vi "NIFPGA-MCS.get bin data.vi"(0 "i ref in":refnum<vi>, 3 "ms timeout (10000)":i32=10000, 5 "error in (no error)":errorcluster) -> (14 "i ref out":refnum<vi>, 16 "Output Waveform":waveform(dbl), 19 "error out":errorcluster)   [LabVIEW 2014, in "NIFPGA-MCS.lvlib"]
doc: "Reads the previously acquired data from the device."
uses:
  NIFPGA-MCS.lvlib
  CSCore/CSApplicationBaseClasses/MCSBase/MCSBase.directionType.ctl
  CSCore/CSApplicationBaseClasses/MCSBase/MCSBase.serviceType.ctl
  CSlibraries/UtilityLib/UtilityLib.valueStatus.ctl
  CSCore/CSApplicationBaseClasses/DeviceBase/DeviceBase.deviceState.ctl
  CSCore/CSSystem/CoreDefs/CoreDefs.error_type.ctl
  CSCore/CSSystem/CoreDefs/CoreDefs.error_severity.ctl
  CSCore/CSApplicationBaseClasses/MCSBase/MCSBase.lvlib
  CSlibraries/UtilityLib/UtilityLib.lvlib
  CSCore/CSApplicationBaseClasses/DeviceBase/DeviceBase.lvlib
  CSCore/CSSystem/CoreLib/CoreLib.lvlib
  CSinstr.lib/NI-FPGA-MCS/host/instrumentDriver/NI-FPGA-MCS_Driver.lvlib
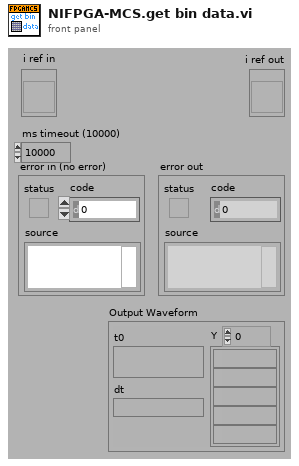
[diagram p1: front panel]
types:
  T1 = typedef "MCSBase.lvlib/MCSBase.serviceType.ctl" = enum16{"counts", "totalCounts", "binWidth", "nOfBins", "nOfRecords", "status", "discrLevel", "discrSlope", "triggerLevel", "triggerSlope"}
  T2 = typedef "UtilityLib.lvlib/UtilityLib.valueStatus.ctl" = enum16{"no info available", "stand by/off", "on", "warning", "alarm/malfunction", "not implemented", "user action required", "important information", "system default", "control default", "indicator default", "button default"}
  T3 = typedef "CoreDefs.error_severity.ctl" = enum16{"undefined", "information", "warning", "error", "fatal"}
  T4 = typedef "CoreDefs.error_type.ctl" = enum16{"no error", "can't load process", "can't unload process", "process does not exist", "can't install process", "can't remove process", "unknown function", "time out", "can't execute function", "duplicate queue name", "super not found", "caller queue invalid", "can't ping process", "unknown error", "VISA Error", "VISA timeout", "GPIB timeout", "GPIB error", "communication error", "data type mismatch", "can't read data from OPC server", "can't write data to OPC server", "OET error", "function not implemented", "process already exists", "invalid Shared Variable name", "error writing Shared Variable", "error reading Shared Variable", "invalid client name", "corrupt database", "unknown class", "call not authorized", "parameter out of range", "OET timeout: can't get data to modify", "invalid queue name", "requested operation incompatible with current state", "event undefined", "event disabled", "state undefined", "caller is not a friend", "EventBuilder: bad eventID", "EventBuilder: no DAQ devices", "a thread must not stop itself", "UNUSED ELEMENT4", "DiscArchiver: eventData incomplete", "DiscArchiver: eventData does not belong to run", "DiscArchiver: can't open file", "DiscArchiver: can't write to file", "DiscArchiver: available disc space low", "can't acquire semaphore", "error reading data from database", "notifier object is not existing", "can't register process", "can't unregister process", "illegal event type", "object disabled", "object already exists", "can't change state", "Instrument not found", "no connection to remote node", "invalid reference", "N/A", "UNUSED ELEMENT 1", "element not found", "illegal TCP/IP connection detected", "object does not exist", "invalid access ID", "unknown CS system", "invalid privilige", "unsupported data type", "unsupported server type", "IO server already exists", "Shared Variable already exists"}
  T5 = typedef "MCSBase.lvlib/MCSBase.directionType.ctl" = enum16{"unknown", "update actual value", "update nominal value", "update both"}
  T6 = typedef "NIFPGA-MCS.lvlib/NIFPGA-MCS.i attribute.ctl" = cluster{"fpgaViRef":T7}
  T7 = typedef "NI-FPGA-MCS_Driver.lvlib/fpga_vi_ref.ctl" = refnum<k20>
  T8 = typedef "MCSBase.lvlib/MCSBase.i attribute.ctl" = cluster{"actValues":T9, "nomValues":T9}
  T9 = typedef "MCSBase.lvlib/MCSBase.parameters.ctl" = cluster{"counts":i32, "totalCounts":i32, "status":i32, "binWidth [us]":dbl, "nOfBins":i32, "nOfRecords":i32, "discLevel [V]":dbl, "discSlope":bool, "triggerLevel [V]":dbl, "triggerSlope":bool, "serviceIDs":cluster{"countslID":i32, "totalCountsID":i32, "binWidthID":i32, "nOfBinsID":i32, "nOfRecordsID":i32, "statusID":i32, "discLevelID":i32, "discSlopeID":i32, "triggerLevelID":i32, "triggerSlopeID":i32}}
  T10 = typedef "DeviceBase.lvlib/DeviceBase.deviceState.ctl" = i16
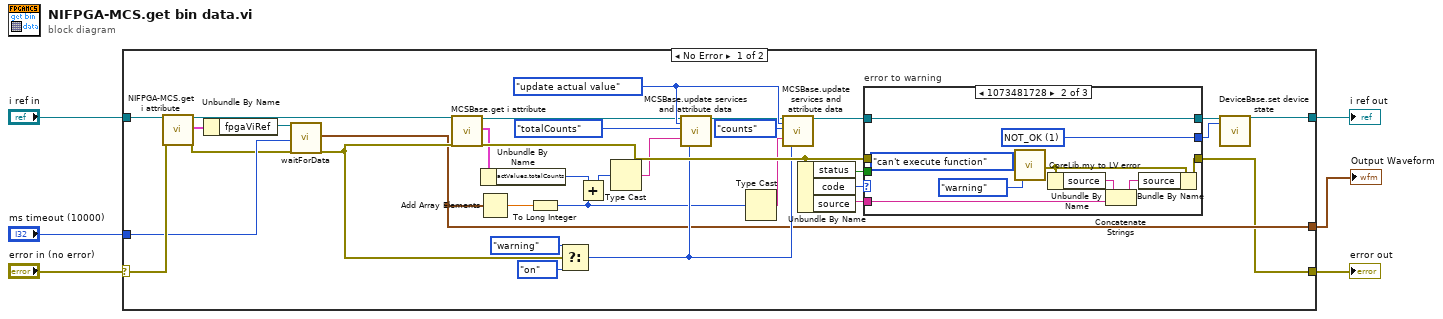
[diagram p0: block diagram]
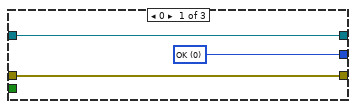
[diagram p2: hidden frame]
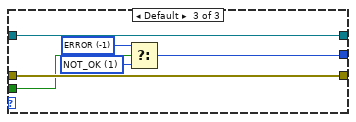
[diagram p3: hidden frame]
diagram:
  n1 = case shown="No Error" "error in (no error)" {
    selector: "error in (no error)" -> [w38 w58]
    tunnel: "i ref in" -> [w39 w59]
    tunnel: [w15 w59] -> w4
    tunnel: [w9 w58] -> w3
    tunnel: "ms timeout (10000)" -> [w13 _]
    tunnel: [w10 _] -> w1
    frame No Error {
      w26 = MCSBase.directionType."update actual value" ("direction")
      n2 = call "NIFPGA-MCS.get i attribute.vi"("i ref in"=w39, "error in (no error)"=w38) -> ("i ref out"=w8:refnum<vi>, "i attribute"=w37:T6, "error out"=w12:errorcluster)  [unwired: 15 in]
      n3 = Unbundle By Name(w37) -> ("fpgaViRef"=w14:T7)
      n4 = call "waitForData.vi"("fpga_vi_ref"=w14, "Timeout (10000) [ms]"=w13, "error in (no error)"=w12) -> ("data"=w10:waveform(dbl), "error out"=w11:errorcluster)  [unwired: 13 in, 2 out]
      n5 = call "MCSBase.get i attribute.vi"("i ref in"=w8, "error in (no error)"=w11) -> ("i ref out"=w19:refnum<vi>, "i attribute"=w16:T8, "error out"=w32:errorcluster)  [unwired: 15 in]
      n6 = Add Array Elements(numeric array=w10) -> (sum=w17:dbl)
      n7 = Unbundle By Name(w16) -> ("actValues.totalCounts"=w18:i32)
      n8 = To Long Integer(number=w17) -> (32bit integer=w28:i32)
      n9 = Select(t=UtilityLib.valueStatus."warning" ("quality"), s=w11, f=UtilityLib.valueStatus."on" ("quality")) -> (s? t:f=w30:T2)
      n10 = Add(x=w18, y=w28) -> (x+y=w21:i32)
      n11 = Type Cast(x=w21) -> (*(type *) &x=w22:string)  [unwired: 1 in]
      n12 = call "MCSBase.update services and attribute data.vi"("i ref in"=w19, "direction"=w26, "service"=MCSBase.serviceType."totalCounts", "value"=w22, "quality"=w30) -> ("i ref out"=w25:refnum<vi>)  [unwired: 12 in, 2 out]
      n13 = Type Cast(x=w28) -> (*(type *) &x=w29:string)  [unwired: 1 in]
      n14 = call "MCSBase.update services and attribute data.vi"("i ref in"=w25, "direction"=w26, "service"=MCSBase.serviceType."counts", "value"=w29, "quality"=w30) -> ("i ref out"=w34:refnum<vi>)  [unwired: 12 in, 2 out]
      n15 = Unbundle By Name(w32) -> ("status"=w7:bool, "code"=w31:i32, "source"=w36:string)
      n16 = case "error to warning" shown="1073481728" w31 {
        tunnel: w32 -> [w42 _ w56]
        tunnel: [w42 w46 w56] -> w9
        tunnel: [w40 w51 w52] -> w33
        tunnel: w34 -> [w41 w50 w57]
        tunnel: [w41 w50 w57] -> w35
        tunnel: w36 -> [_ w43 _]
        tunnel: w7 -> [_ _ w55]
        frame 0 {
          w40 = T10 0 items=["ERROR"=-1, "OK"=0, "NOT_OK"=1] ("deviceState")
        }
        frame 1073481728 {
          w51 = T10 1 items=["ERROR"=-1, "OK"=0, "NOT_OK"=1] ("deviceState")
          n17 = call "CoreLib.my to LV error.vi"("ErrorTypes"=CoreDefs.error_type."can't execute function", "severityLevel"=CoreDefs.error_severity."warning") -> ("myErrorCluster"=w47:errorcluster)  [unwired: 16 in, 1 out]
          n18 = Unbundle By Name(w47) -> ("source"=w45:string)
          n19 = Concatenate Strings(w45, w43) -> (w44:string)
          n20 = Bundle By Name(cluster=w47, "source"=w44) -> (w46:errorcluster)
        }
        frame Default {
          w53 = T10 1 items=["ERROR"=-1, "OK"=0, "NOT_OK"=1] ("f")
          w54 = T10 -1 items=["ERROR"=-1, "OK"=0, "NOT_OK"=1] ("deviceState")
          n21 = Select(t=w54, s=w55, f=w53) -> (s? t:f=w52:T10)
        }
      }
      n22 = call "DeviceBase.set device state.vi"("i ref in"=w35, "deviceState"=w33) -> ("i ref out"=w15:refnum<vi>)  [unwired: 15 in, 2 out]
    }
    frame Error {
    }
  }
  "error out" <- w3
  "i ref out" <- w4
  "Output Waveform" <- w1
